vi "File Viewer.vi"() -> ()   [LabVIEW 2019]
uses:
  <vilib>/Utility/file.llb/Read Delimited Spreadsheet (I64).vi
panel:
  in  "?":bool
  in  "Tab Control":T1(tab)
  out "Raw Image From Camera":i32[][](graph)
  in  "file path for picture":path
  out "Expected position on spectrometer (pixels):":dbl
  in  "Grating:":u16(ring) items=["Shimadzu 30-006  "]
  in  "Laser:":u16(ring) items=["800nm  "]
  in  "Harmonic":dbl min=10.0 max=40.0
  out "l (nm)":dbl
  out "E (J)":dbl
  out "E (eV)":dbl
  out "Nearest Harmonic of 800nm":dbl
  out "Vertical Binned Waveform Graph":i64[](graph)
  out "Cursor Position (pixels)":dbl
  out "Distance to nearest harmonic of 800nm (pixels)":dbl
  in  "Caibration Date":u16(ring) items=["first calibration - 7/31", "7/31-current"]
  out "Wavelength Graph":cluster{"lamda (m)":dbl, "Numeric":i64}[](graph)
  out "Energy Graph (eV)":cluster{"lamda (m)":dbl, "Numeric":i64}[](graph)
  out "Harmonics Graph":cluster{"lamda (m)":dbl, "Numeric":i64}[](graph)
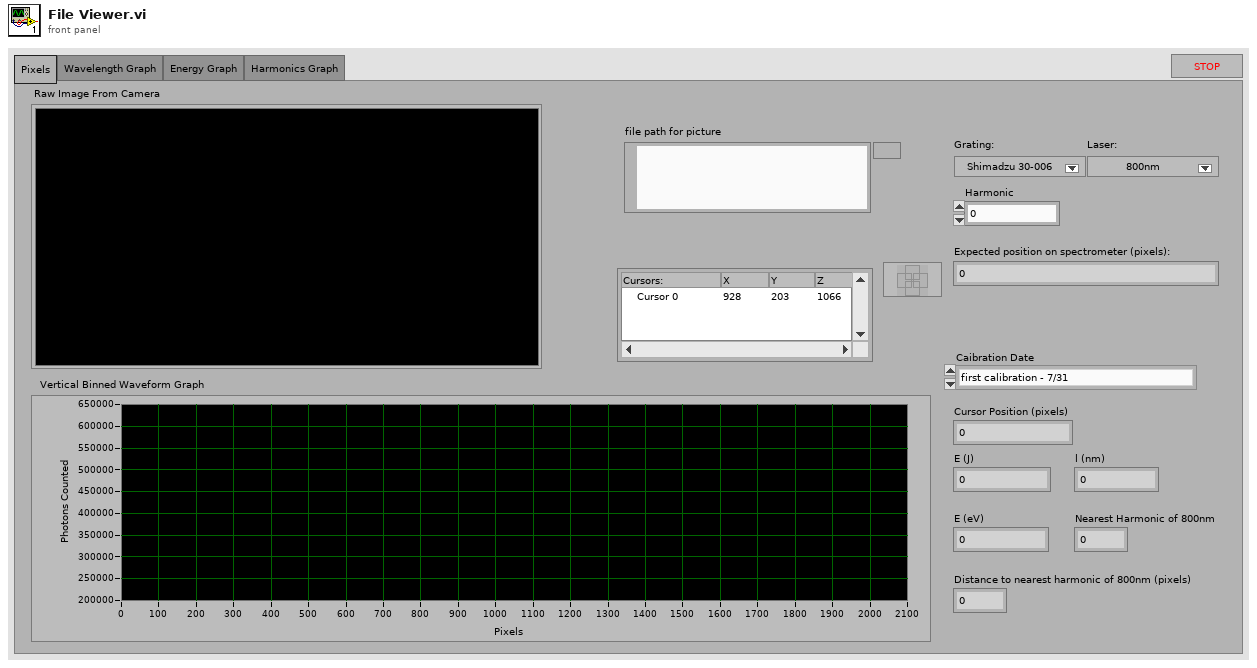
[diagram p1: front panel]
types:
  T1 = enum32{"Pixels", "Wavelength Graph", "Energy Graph", "Harmonics Graph"}
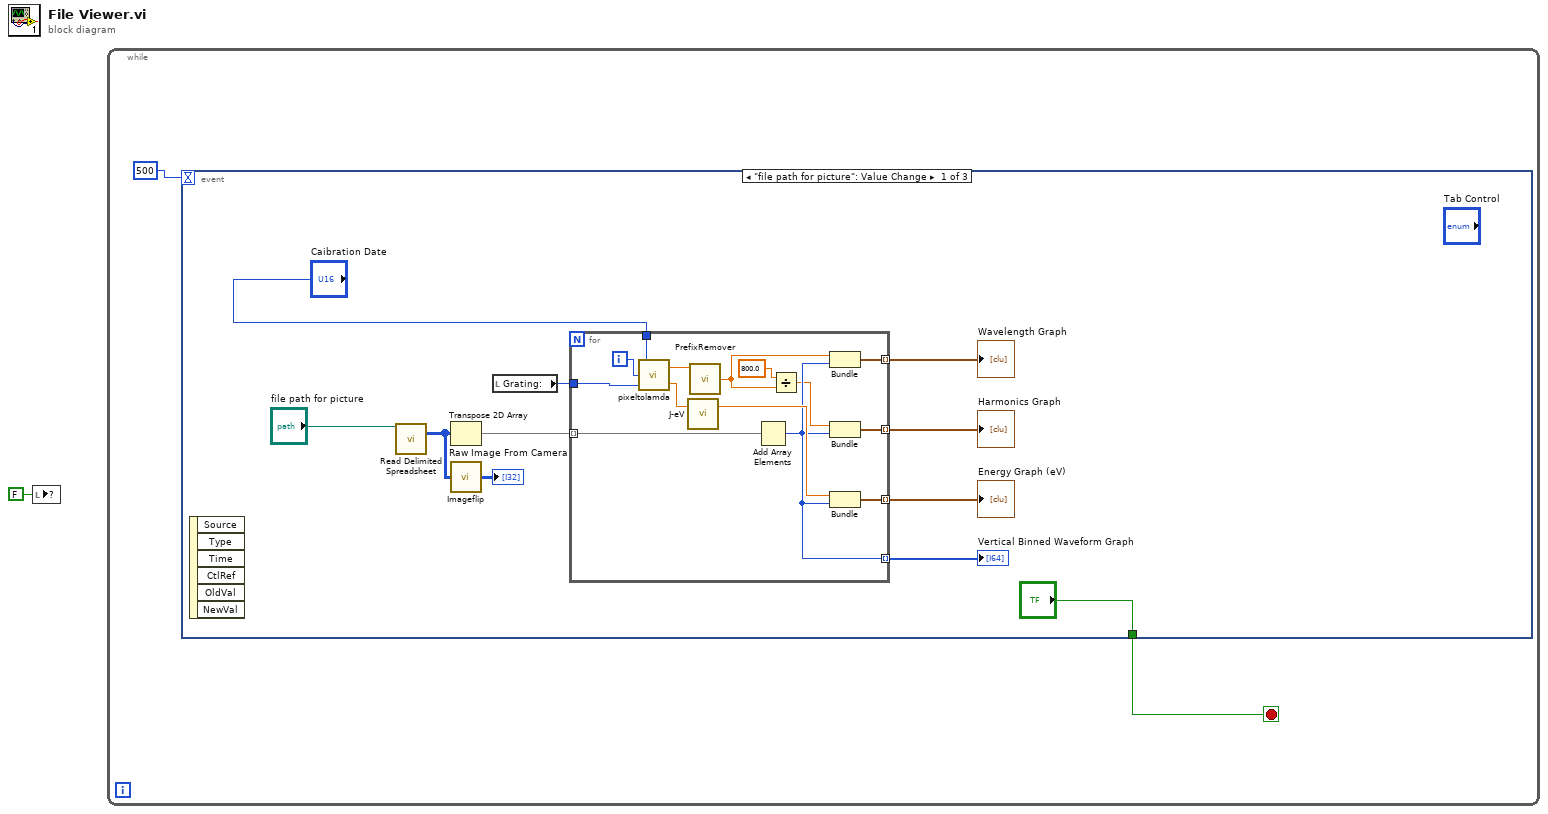
[diagram p0: block diagram]
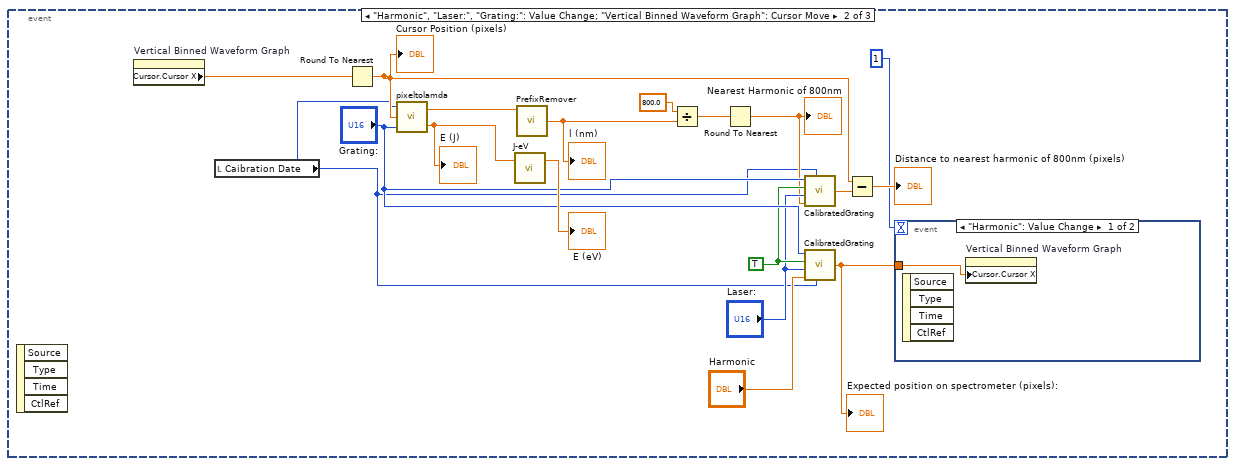
[diagram p2: hidden frame]
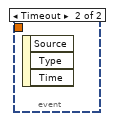
[diagram p3: hidden frame]
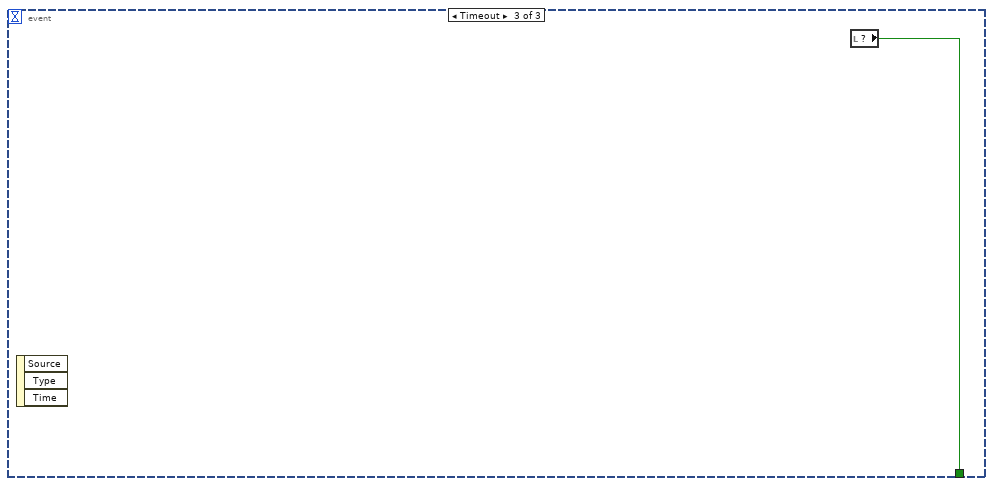
[diagram p4: hidden frame]
diagram:
  n1 = local write item#1(FALSE) -> ()
  n2 = while {
    stop <- w3 stop-if-true
    n3 = event shown="[0] \"file path for picture\": Value Change" {
      selector: _ -> [_ _ _]
      dyn-events: _ -> [_ _ _]
      timeout: 500 -> [_ _ _]
      tunnel: ["?" _ w48] -> w3
      event "file path for picture": Value Change {
        n4 = event-data() -> ()  [unwired: 1 in, 6 out]
        n5 = call-poly <vilib>:"Read Delimited Spreadsheet.vi"("file path (dialog if empty)"="file path for picture") -> ("all rows"=w11:i64[][])  [unwired: 9 in, 5 out]
        n6 = Transpose 2D Array(2D array=w11) -> (transposed array=w10:i64[][])
        n7 = call "Imageflip.vi"("2D array"=w11) -> ("transposed array"=→"Raw Image From Camera":i32[][])
        n8 = local read "Grating:"() -> (w8:u16)
        n9 = for {
          tunnel: w10 -> [w28] mode=indexing
          tunnel: [w21] -> w9 mode=indexing
          tunnel: w8 -> [w26]
          tunnel: [w25] -> w7 mode=indexing
          tunnel: [w22] -> w6 mode=indexing
          tunnel: [w16] -> w5 mode=indexing
          tunnel: "Caibration Date" -> [w15]
          i -> [w27]
          n10 = call "pixeltolamda.vi"("Grating:"=w26, "Pixel Postion"=w27, "Caibration Date"=w15) -> ("E (J)"=w24:dbl, "lamda (m)"=w19:dbl)
          n11 = call "J-eV.vi"("J"=w24) -> ("eV"=w23:dbl)  [unwired: 1 in, 1 out]
          n12 = call "PrefixRemover.vi"("Nano"=w19) -> ("No prefix"=w18:dbl)  [unwired: 3 in]
          n13 = Add Array Elements(numeric array=w28) -> (sum=w21:i64)
          n14 = Divide(x=800.0, y=w18) -> (x/y=w17:dbl)
          n15 = Bundle("No prefix"=w18, "Numeric"=w21) -> (w25:cluster{"No prefix":dbl, "Numeric":i64})  [unwired: 1 in]
          n16 = Bundle(w17, "Numeric"=w21) -> (w16:cluster{dbl, "Numeric":i64})  [unwired: 1 in]
          n17 = Bundle("eV"=w23, "Numeric"=w21) -> (w22:cluster{"eV":dbl, "Numeric":i64})  [unwired: 1 in]
        }
        "Vertical Binned Waveform Graph" <- w9
        "Wavelength Graph" <- w7
        "Energy Graph (eV)" <- w6
        "Harmonics Graph" <- w5
      }
      event "Harmonic", "Laser:", "Grating:": Value Change; "Vertical Binned Waveform Graph": Cursor Move {
        w38 = TRUE ("Subvi?")
        n18 = event-data() -> ()  [unwired: 1 in, 4 out]
        n19 = property on="Vertical Binned Waveform Graph" class="WFGraph (strict)"() -> ("Cursor.Cursor X"=w40:dbl)  [unwired: 2 in, 2 out]
        n20 = local read "Caibration Date"() -> (w29:u16)
        n21 = Round To Nearest(number=w40) -> (nearest integer value=w32:dbl)
        "Cursor Position (pixels)" <- w32
        n22 = call "pixeltolamda.vi"("Grating:"="Grating:", "Pixel Postion"=w32, "Caibration Date"=w29) -> ("E (J)"=w44:dbl, "lamda (m)"=w45:dbl)
        "E (J)" <- w44
        n23 = call "J-eV.vi"("J"=w44) -> ("eV"=→"E (eV)":dbl)  [unwired: 1 in, 1 out]
        n24 = call "PrefixRemover.vi"("Nano"=w45) -> ("No prefix"=w35:dbl)  [unwired: 3 in]
        "l (nm)" <- w35
        n25 = Divide(x=800.0, y=w35) -> (x/y=w42:dbl)
        n26 = Round To Nearest(number=w42) -> (nearest integer value=w36:dbl)
        "Nearest Harmonic of 800nm" <- w36
        n27 = call "CalibratedGrating.vi"("Grating:"="Grating:", "Subvi?"=w38, "Laser:"="Laser:", "Harmonic"=w36, "Caibration Date"=w29) -> ("Position on spectrometer (pixels):"=w34:dbl)
        n28 = call "CalibratedGrating.vi"("Grating:"="Grating:", "Subvi?"=w38, "Laser:"="Laser:", "Harmonic"="Harmonic", "Caibration Date"=w29) -> ("Position on spectrometer (pixels):"=w31:dbl)
        "Expected position on spectrometer (pixels):" <- w31
        n29 = Subtract(x=w32, y=w34) -> (x-y=→"Distance to nearest harmonic of 800nm (pixels)":dbl)
        n30 = event shown="[0] \"Harmonic\": Value Change" {
          selector: _ -> [_ _]
          dyn-events: _ -> [_ _]
          timeout: 1 -> [_ _]
          tunnel: w31 -> [w47 _]
          event "Harmonic": Value Change {
            n31 = event-data() -> ()  [unwired: 1 in, 4 out]
            n32 = property on="Vertical Binned Waveform Graph" class="WFGraph (strict)"("Cursor.Cursor X"=w47) -> ()  [unwired: 2 in, 2 out]
          }
          event Timeout {
            n33 = event-data() -> ()  [unwired: 1 in, 3 out]
          }
        }
      }
      event Timeout {
        n34 = event-data() -> ()  [unwired: 1 in, 3 out]
        n35 = local read item#1() -> (w48:bool)
      }
    }
  }
